vi "Write_Reg (SubVI).vi"(8 "error in (no error)":errorcluster, 9 "data in":string, 11 "TCP Network Connection in":refnum<k5>) -> (0 "error out":errorcluster, 1 "data out":string, 3 "TCP Network Connection out":refnum<k5>)   [LabVIEW 2019]
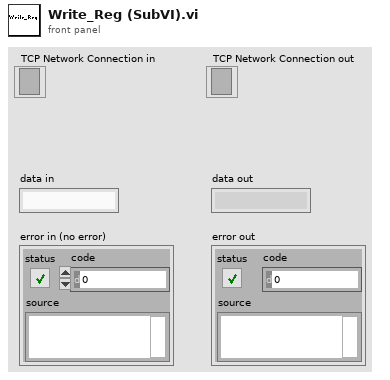
[diagram p1: front panel]
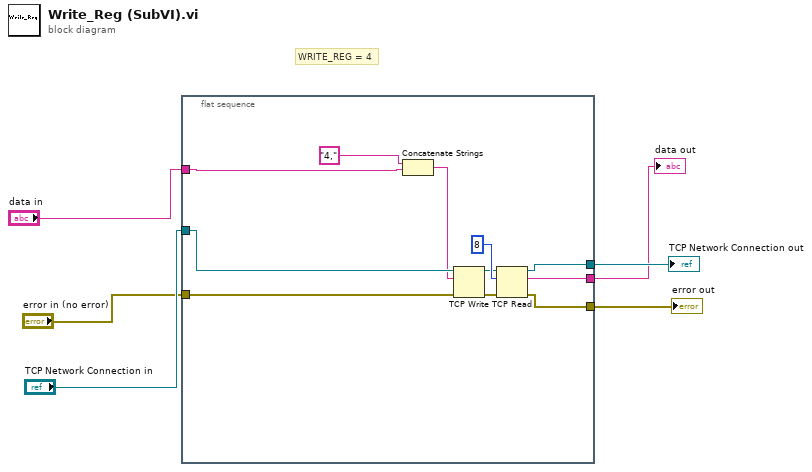
[diagram p0: block diagram]
diagram:
  # "WRITE_REG = 4"
  n1 = flat-sequence {
    tunnel: "TCP Network Connection in" -> [w17]
    tunnel: "error in (no error)" -> [w16]
    tunnel: "data in" -> [w11]
    tunnel: [w9] -> w3
    tunnel: [w8] -> w2
    tunnel: [w7] -> w1
    frame #0 {
      n2 = Concatenate Strings("4," ("data in"), w11) -> (w10:string)
      n3 = TCP Write(connection ID=w17, data in=w10, error in (no error)=w16) -> (connection ID out=w14:refnum<k5>, error out=w13:errorcluster)  [unwired: 1 in, 1 out]
      n4 = TCP Read(connection ID=w14, bytes to read=8, error in (no error)=w13) -> (connection ID out=w8:refnum<k5>, data out=w7:string, error out=w9:errorcluster)  [unwired: 2 in]
    }
  }
  "error out" <- w3
  "TCP Network Connection out" <- w2
  "data out" <- w1
